vi "From Service.vi"(11 "Entity Manager Service":refnum<class "Entity Manager Service.lvclass">) -> (3 "Entity Manager":refnum<class "Entity Manager.lvclass">)   [LabVIEW 2020, in "HTTP-Conditum.lvlib" / "Entity Manager Service.lvclass"]
uses:
  Entity Manager Service.lvclass
  <vilib>/IlluminatedG/IG Conditum/Conditum/Entity Manager/Entity Manager.lvclass
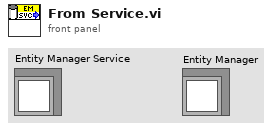
[diagram p1: front panel]
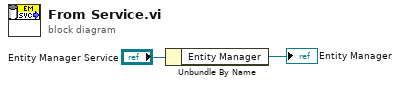
[diagram p0: block diagram]
diagram:
  n1 = Unbundle By Name("Entity Manager Service") -> ("Entity Manager"=→"Entity Manager":refnum<class "Entity Manager.lvclass">)
